vi "Labview2010ExampleForOceanDirect.vi"() -> ()   [LabVIEW 2010]
uses:
  C:/Program Files/Ocean Insight/OceanDirect SDK/lib/NetOceanDirect.dll
  Program Files/Ocean Insight/OceanDirect SDK/lib/NetOceanDirect.dll
panel:
  in  "Integration time (us)":u32=10000
  in  "Use this stop button and not the LabVIEW abort button to allow clean up code to be exicuted":bool
  out "Spectrum":T1(graph)
  # "Simple demostration of using OceanDirect in LabVIEW via the .NET interface"
  # "See back panel for details on how to set up this deomonstration"
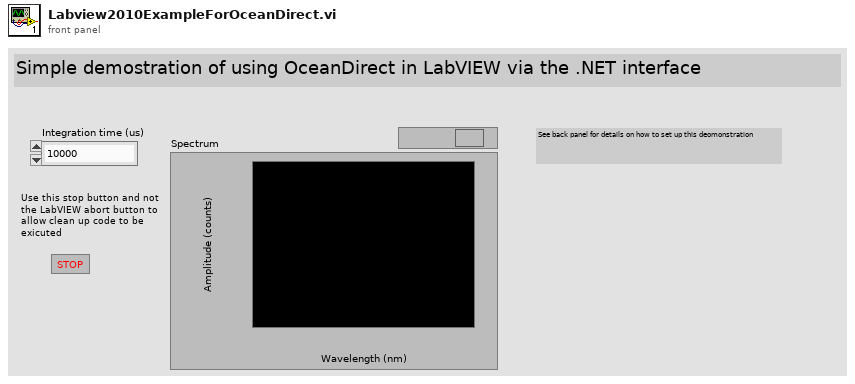
[diagram p1: front panel]
types:
  T1 = cluster{"getWavelengths":dbl[], "getSpectrum":dbl[]}
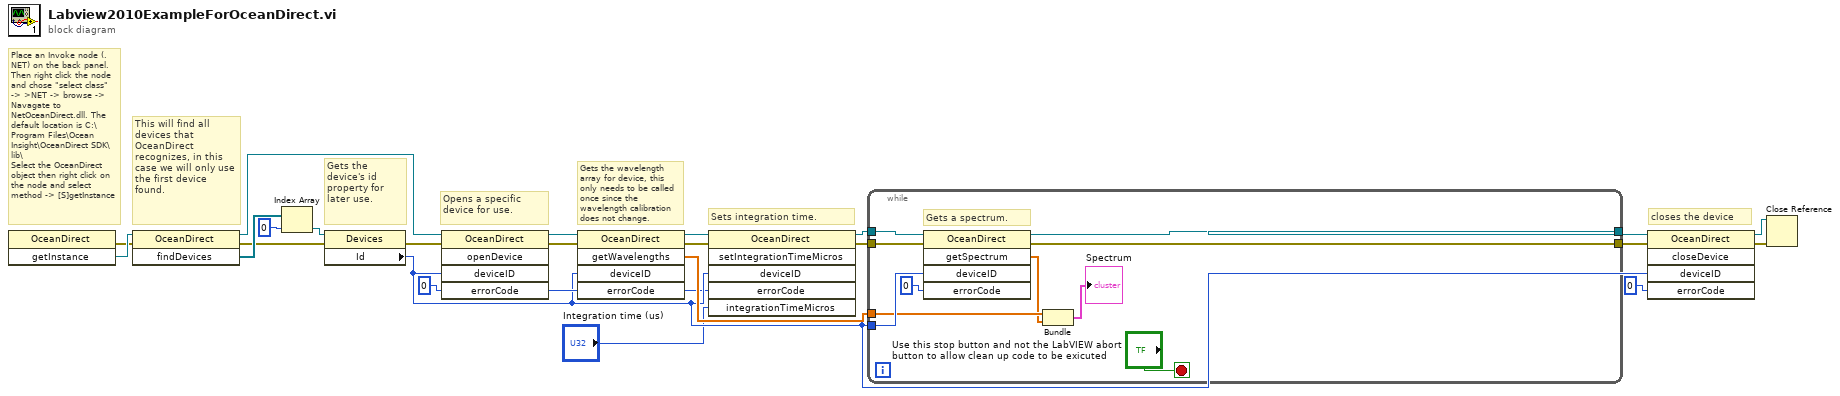
[diagram p0: block diagram]
diagram:
  # "closes the device"
  # "Place an Invoke node (.NET) on the back panel. Then right click the node and chose \"select class\" -> >NET -> browse -> Navagate to NetOceanDirect.dll. The default location is C:\\Program Files\\Ocean Insight\\OceanDirect SDK\\lib\\\nSelect the OceanDirect object then right click on the node and select method -> [S]getInstance"
  # "Sets integration time."
  # "Gets the wavelength array for device, this only needs to be called once since the wavelength calibration does not change."
  # "Opens a specific device for use."
  # "Gets the device's id property for later use."
  # "This will find all devices that OceanDirect recognizes, in this case we will only use the first device found."
  n1 = invoke class="OceanDirect" method="getInstance"() -> (error out=w10:errorcluster, "getInstance"=w11:refnum<k24>)  [unwired: 3 in, 1 out]
  n2 = invoke class="OceanDirect" method="findDevices"(reference=w11, error in=w10) -> (reference out=w18:refnum<k24>, error out=w15:errorcluster, "findDevices"=w25:refnum<k24>[])  [unwired: 1 in]
  n3 = Index Array(array=w25, index=0) -> (element=w23:refnum<k24>)
  n4 = property class="Devices"(reference=w23, error in=w15) -> (error out=w14:errorcluster, "Id"=w8:i32)  [unwired: 1 out]
  n5 = invoke class="OceanDirect" method="openDevice"(reference=w18, error in=w14, "deviceID"=w8, "errorCode"=0) -> (reference out=w12:refnum<k24>, error out=w3:errorcluster, "errorCode"=w13:i32)  [unwired: 1 in, 2 out]
  n6 = invoke class="OceanDirect" method="getWavelengths"(reference=w12, error in=w3, "deviceID"=w8, "errorCode"=w13) -> (reference out=w4:refnum<k24>, error out=w5:errorcluster, "getWavelengths"=w9:dbl[], "errorCode"=w7:i32)  [unwired: 1 in, 1 out]
  n7 = invoke class="OceanDirect" method="setIntegrationTimeMicros"(reference=w4, error in=w5, "deviceID"=w8, "errorCode"=w7, "integrationTimeMicros"="Integration time (us)") -> (reference out=w2:refnum<k24>, error out=w1:errorcluster)  [unwired: 1 in, 4 out]
  n8 = while {
    tunnel: [w34] -> w20
    tunnel: w8 -> [w33]
    tunnel: w9 -> [w29]
    tunnel: w2 -> [w32]
    tunnel: [w31] -> w17
    tunnel: w1 -> [w26]
    stop <- "Use this stop button and not the LabVIEW abort button to allow clean up code to be exicuted" stop-if-true
    # "Gets a spectrum."
    n9 = invoke class="OceanDirect" method="getSpectrum"(reference=w32, error in=w26, "deviceID"=w33, "errorCode"=0) -> (reference out=w31:refnum<k24>, error out=w34:errorcluster, "getSpectrum"=w28:dbl[])  [unwired: 1 in, 2 out]
    n10 = Bundle("getWavelengths"=w29, "getSpectrum"=w28) -> (→"Spectrum":T1)  [unwired: 1 in]
  }
  n11 = invoke class="OceanDirect" method="closeDevice"(reference=w17, error in=w20, "deviceID"=w8, "errorCode"=0) -> (reference out=w16:refnum<k24>, error out=w21:errorcluster)  [unwired: 1 in, 3 out]
  n12 = Close Reference(reference=w16, error in (no error)=w21) -> ()  [unwired: 1 out]
